vi "Handle Video Image.vi"(4 "queue in":refnum<queue>, 5 "Event Data":cluster{"sender":refnum<k24>, "e":refnum<k24>}, 6 "Control Ref":refnum<k24>, 7 "Event Common Data":T1) -> ()   [LabVIEW 2010, in "Kinect_API.lvlib"]
uses:
  Kinect_API.lvlib
  Microsoft.Research.Kinect
  <vilib>/vision/Image Controls.llb/IMAQ Image.ctl
  <vilib>/vision/NI_Vision_Development_Module.lvlib
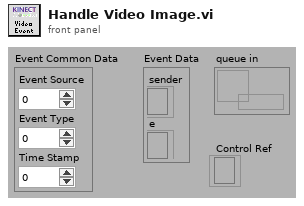
[diagram p1: front panel]
types:
  T1 = cluster{"Event Source":i32, "Event Type":u32, "Time Stamp":u32}
  T2 = typedef "Image Type" = u32
  T3 = typedef "IMAQ Image.ctl" = refnum<image>
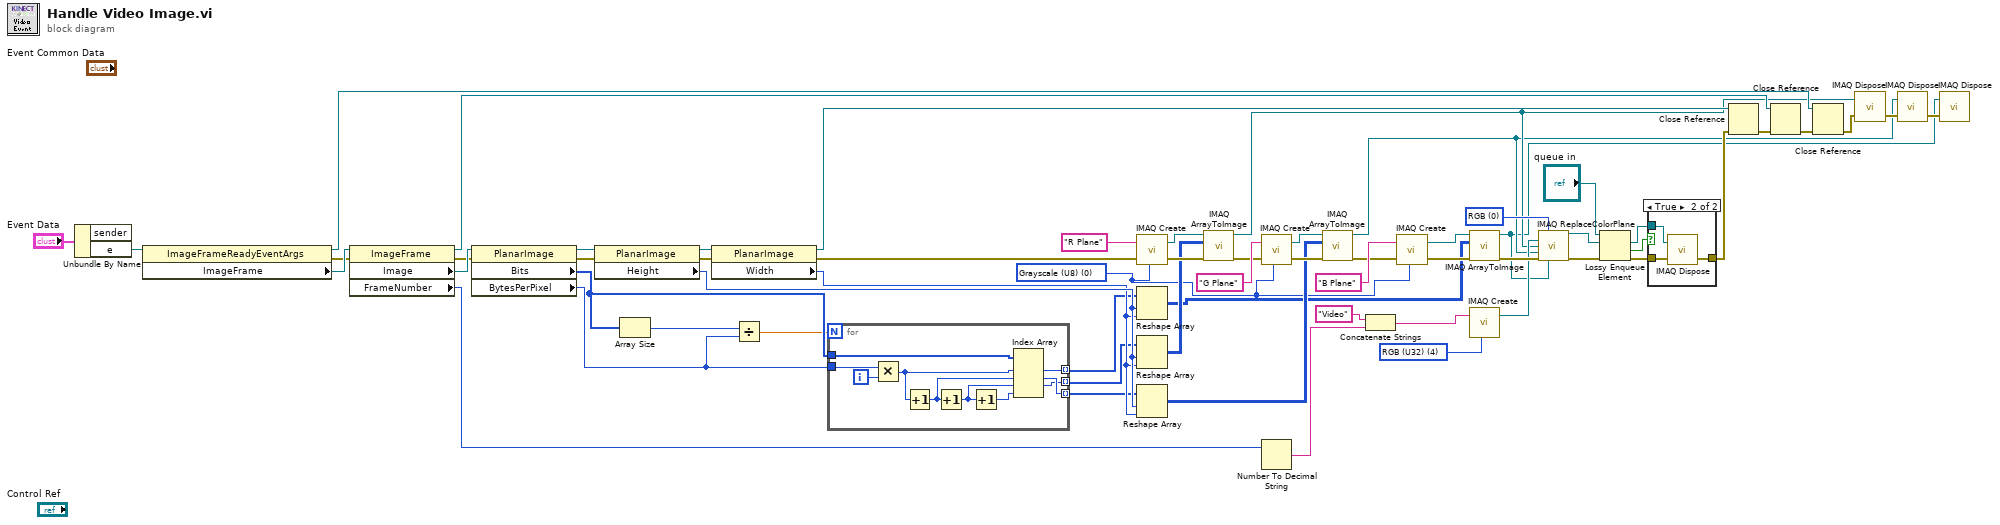
[diagram p0: block diagram]
diagram:
  w13 = T2 4 items=["Grayscale (U8)", "Grayscale (I16)", "Grayscale (SGL)", "Complex (CSG)", "RGB (U32)", "HSL (U32)", "RGB (U64)", "Grayscale (U16)"] ("Image Type")
  w14 = T2 0 items=["Grayscale (U8)", "Grayscale (I16)", "Grayscale (SGL)", "Complex (CSG)", "RGB (U32)", "HSL (U32)", "RGB (U64)", "Grayscale (U16)"] ("Image Type")
  w37 = u16 0 items=["RGB", "HSL", "HSV", "HSI"] ("Color Mode")
  n1 = Unbundle By Name("Event Data") -> ("e"=w61:refnum<k24>)  [unwired: 1 out]
  n2 = property class="ImageFrameReadyEventArgs"(reference=w61) -> (reference out=w50:refnum<k24>, error out=w47:errorcluster, "ImageFrame"=w60:refnum<k24>)  [unwired: 1 in]
  n3 = property class="ImageFrame"(reference=w60, error in=w47) -> (reference out=w51:refnum<k24>, error out=w48:errorcluster, "Image"=w54:refnum<k24>, "FrameNumber"=w18:i32)
  n4 = property class="PlanarImage"(reference=w54, error in=w48) -> (reference out=w57:refnum<k24>, error out=w59:errorcluster, "Bits"=w33:u8[], "BytesPerPixel"=w30:i32)
  n5 = property class="PlanarImage"(reference=w57, error in=w59) -> (reference out=w55:refnum<k24>, error out=w58:errorcluster, "Height"=w29:i32)
  n6 = Array Size(array=w33) -> (size(s)=w32:i32)
  n7 = property class="PlanarImage"(reference=w55, error in=w58) -> (reference out=w56:refnum<k24>, error out=w11:errorcluster, "Width"=w28:i32)
  n8 = Divide(x=w32, y=w30) -> (x/y=w31:dbl)
  n9 = for {
    N: w31 -> [_]
    tunnel: w33 -> [w66]
    tunnel: [w65] -> w22 mode=indexing
    tunnel: [w64] -> w27 mode=indexing
    tunnel: [w63] -> w23 mode=indexing
    tunnel: w30 -> [w62]
    i -> [w71]
    n10 = Multiply(x=w62, y=w71) -> (x*y=w70:i32)
    n11 = Increment(x=w70) -> (x+1=w69:i32)
    n12 = Increment(x=w69) -> (x+1=w68:i32)
    n13 = Increment(x=w68) -> (x+1=w67:i32)
    n14 = Index Array(array=w66, index #1=w70, index #2=w69, index #3=w68, index #4=w67) -> (element #1=w65:u8, element #2=w64:u8, element #3=w63:u8)  [unwired: 1 out]
  }
  n15 = call "IMAQ Create"("Image Name"="R Plane", "Image Type"=w14, "error in (no error)"=w11) -> ("New Image"=w44:T3, "error out"=w43:errorcluster)  [unwired: 2 in]
  n16 = Reshape Array(w22, w29, w28) -> (w24:u8[][])
  n17 = Reshape Array(w23, w29, w28) -> (w26:u8[][])
  n18 = Reshape Array(w27, w29, w28) -> (w25:u8[][])
  n19 = call "IMAQ ArrayToImage"("error in (no error)"=w43, "Image Pixels (U8)"=w26, "Image"=w44) -> ("error out"=w36:errorcluster, "Image Out"=w3:T3)  [unwired: 7 in]
  n20 = call "IMAQ Create"("Image Name"="G Plane", "Image Type"=w14, "error in (no error)"=w36) -> ("New Image"=w45:T3, "error out"=w46:errorcluster)  [unwired: 2 in]
  n21 = Number To Decimal String(number=w18) -> (decimal integer string=w17:string)  [unwired: 1 in]
  n22 = call "IMAQ ArrayToImage"("error in (no error)"=w46, "Image Pixels (U8)"=w25, "Image"=w45) -> ("error out"=w35:errorcluster, "Image Out"=w2:T3)  [unwired: 7 in]
  n23 = Concatenate Strings("Video" ("string"), w17) -> (w16:string)
  n24 = call "IMAQ Create"("Image Name"="B Plane", "Image Type"=w14, "error in (no error)"=w35) -> ("New Image"=w42:T3, "error out"=w41:errorcluster)  [unwired: 2 in]
  n25 = call "IMAQ ArrayToImage"("error in (no error)"=w41, "Image Pixels (U8)"=w24, "Image"=w42) -> ("error out"=w34:errorcluster, "Image Out"=w1:T3)  [unwired: 7 in]
  n26 = call "IMAQ Create"("Image Name"=w16, "Image Type"=w13) -> ("New Image"=w19:T3)  [unwired: 3 in, 1 out]
  n27 = call "IMAQ ReplaceColorPlane"("Color Mode"=w37, "Image Dst"=w19, "Red or Hue Plane"=w3, "Green or Sat Plane"=w2, "error in (no error)"=w34, "Blue or Luma or Val or Inten Plane"=w1) -> ("Image Dst Out"=w21:T3, "error out"=w20:errorcluster)  [unwired: 8 in]
  n28 = Lossy Enqueue Element(queue="queue in", element=w21, error in (no error)=w20) -> (overflow element=w10:T3, overflow?=w7:bool, error out=w9:errorcluster)  [unwired: 1 out]
  n29 = case shown="True" w7 {
    tunnel: w10 -> [_ w75]
    tunnel: w9 -> [w72 w74]
    tunnel: [w72 w73] -> w8
    frame False {
    }
    frame True {
      n30 = call "IMAQ Dispose"("Image"=w75, "error in (no error)"=w74) -> ("error out"=w73:errorcluster)  [unwired: 4 in]
    }
  }
  n31 = Close Reference(reference=w56, error in (no error)=w8) -> (error out=w53:errorcluster)
  n32 = Close Reference(reference=w51, error in (no error)=w53) -> (error out=w52:errorcluster)
  n33 = Close Reference(reference=w50, error in (no error)=w52) -> (error out=w6:errorcluster)
  n34 = call "IMAQ Dispose"("Image"=w3, "error in (no error)"=w6) -> ("error out"=w5:errorcluster)  [unwired: 4 in]
  n35 = call "IMAQ Dispose"("Image"=w2, "error in (no error)"=w5) -> ("error out"=w4:errorcluster)  [unwired: 4 in]
  n36 = call "IMAQ Dispose"("Image"=w1, "error in (no error)"=w4) -> ()  [unwired: 4 in, 1 out]
